vi "simplification.vi"(3 "jd":dbl, 4 "c":dbl, 5 "jb":dbl, 6 "a":dbl) -> (0 "z":dbl, 1 "jy":dbl, 2 "x":dbl)   [LabVIEW 2013]
panel:
  # "+"
  # "+"
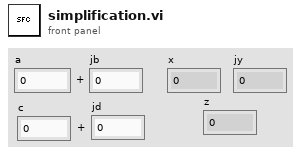
[diagram p1: front panel]
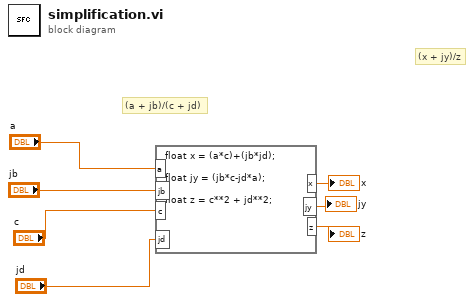
[diagram p0: block diagram]
diagram:
  # "(a + jb)/(c + jd)"
  # "(x + jy)/z"
  n1 = formula code="float x = (a*c)+(jb*jd);\n\nfloat jy = (jb*c-jd*a);\n\nfloat z = c**2 + jd**2;"("a"="a", "jb"="jb", "c"="c", "jd"="jd") -> ("x"=→"x":dbl, "jy"=→"jy":dbl, "z"=→"z":dbl)
